vi "Deactivate.vi"(8 "error in (no error)":errorcluster, 11 "Abstract License in":refnum<class "Software License Manager.lvclass">) -> (0 "error out":errorcluster, 1 "ok?":bool, 3 "Abstract License out":refnum<class "Software License Manager.lvclass">)   [LabVIEW 2021, in "Software License Manager.lvclass"]
uses:
  Software License Manager.lvclass
  Software License Manager.lvclass/Software License Manager.ctl
  Board/Board.lvclass/Board.ctl
  Board/Read Product ID.vi
  Board/Read Host Name.vi
  <vilib>/httpClient/POSTBuffer.vi
  <vilib>/httpClient/LabVIEWHTTPClient.lvlib
  Board/Board.lvclass
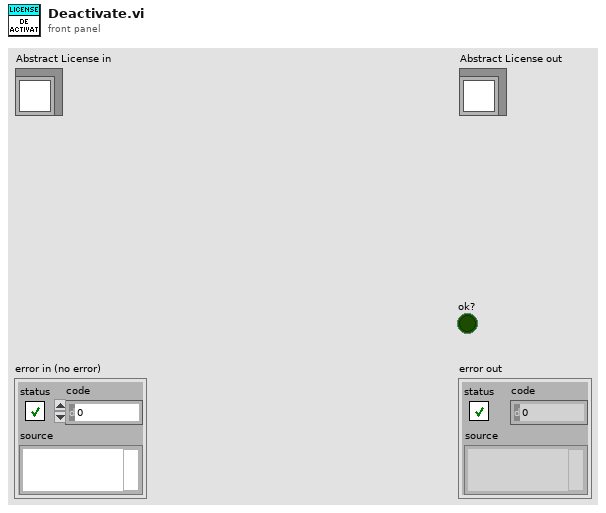
[diagram p1: front panel]
types:
  T1 = typedef "LabVIEWHTTPClient.lvlib/ClientHandle.ctl" = refnum<k1>
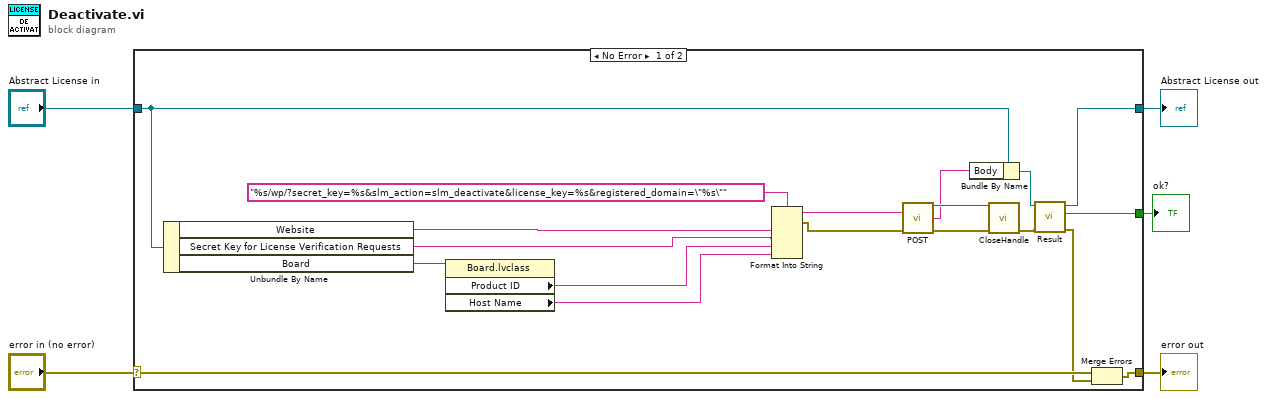
[diagram p0: block diagram]
diagram:
  n1 = case shown="No Error" "error in (no error)" {
    selector: "error in (no error)" -> [w24 w26]
    tunnel: [w16 w26] -> w4
    tunnel: [w11 w25] -> w2
    tunnel: "Abstract License in" -> [w15 w25]
    tunnel: [w7 _] -> w1
    frame No Error {
      n2 = Unbundle By Name(w15) -> ("Website"=w8:string, "Secret Key for License Verification Requests"=w6:string, "Board"=w20:refnum<class "Board.lvclass">)
      n3 = property class="Board.lvclass"(reference=w20) -> ("Product ID"=w9:string, "Host Name"=w10:string)  [unwired: 1 in, 2 out]
      n4 = Format Into String(format string="%s/wp/?secret_key=%s&slm_action=slm_deactivate&license_key=%s&registered_domain=\"%s\"", w8, w6, w9, w10) -> (resulting string=w18:string, error out=w17:errorcluster)  [unwired: 2 in]
      n5 = call-poly <vilib>:"POST.vi"("url"=w18, "error in (no error)"=w17) -> ("client handle out"=w23:T1, "body"=w21:string, "error out"=w22:errorcluster)  [unwired: 10 in, 1 out]
      n6 = Bundle By Name(cluster=w15, "Body"=w21) -> (w12:refnum<class "Software License Manager.lvclass">)
      n7 = call <vilib>:"CloseHandle.vi"("client handle"=w23, "error in (no error)"=w22) -> ("error out"=w14:errorcluster)  [unwired: 13 in]
      n8 = call-dynamic "Result.vi"("error in (no error)"=w14, "Software License Manager in"=w12) -> ("error out"=w13:errorcluster, "ok?"=w7:bool, "Software License Manager out"=w11:refnum<class "Software License Manager.lvclass">)  [unwired: 6 in, 1 out]
      n9 = Merge Errors(w24, w13) -> (w16:errorcluster)
    }
    frame Error {
    }
  }
  "error out" <- w4
  "Abstract License out" <- w2
  "ok?" <- w1
